vi "Write configuration.vi"(8 "error in (no error)":errorcluster, 11 "TomoConversion in":refnum<class "TomoConversion.lvclass">) -> (0 "error out":errorcluster, 3 "TomoConversion out":refnum<class "TomoConversion.lvclass">)   [LabVIEW 2012]
doc: "Writes the configuration cluster into the configuration file. Configuration file is XML-based. It's name is <component ID>.xml"
uses:
  <vilib>/Distrio/Murmex/Murmex/Murmex.lvclass
  TomoConversion.lvclass
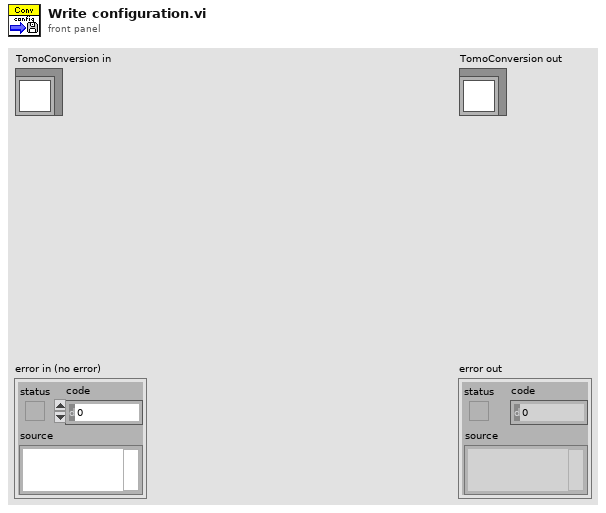
[diagram p1: front panel]
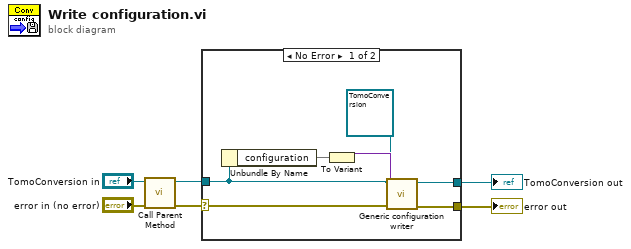
[diagram p0: block diagram]
diagram:
  n1 = call-parent "Call Parent Method"("error in (no error)"="error in (no error)", "Murmex in"="TomoConversion in") -> ("error out"=w4:errorcluster, "Murmex out"=w3:refnum<class "TomoConversion.lvclass">)  [unwired: 8 in]
  n2 = case shown="No Error" w4 {
    selector: w4 -> [w12 w14]
    tunnel: w3 -> [w9 w15]
    tunnel: [w8 w15] -> w2
    tunnel: [w7 w14] -> w1
    frame No Error {
      n3 = Unbundle By Name(w9) -> ("configuration"=w13)
      n4 = To Variant(anything=w13) -> (Variant=w11:variant)
      n5 = call <vilib>:"Generic configuration writer.vi"("error in (no error)"=w12, 9:w11, 10:refnum<class "TomoConversion.lvclass"> refnum ("TomoConversion.lvclass"), "Murmex in"=w9) -> ("error out"=w7:errorcluster, "Murmex out"=w8:refnum<class "TomoConversion.lvclass">)  [unwired: 6 in]
    }
    frame Error {
    }
  }
  "error out" <- w1
  "TomoConversion out" <- w2
